vi "Register PVs.vi"(8 "error in (no error)":errorcluster, 10 "Register Info":T1, 11 "CS++PVMonitor in":refnum<class "CS++PVMonitor.lvclass">) -> (0 "error out":errorcluster, 3 "CS++PVMonitor out":refnum<class "CS++PVMonitor.lvclass">)   [LabVIEW 2015, in "CS++PVMonitor.lvlib" / "CS++PVMonitor.lvclass"]
doc: "Register value change monitoring for process variables."
uses:
  CS++PVMonitor.lvclass
  <vilib>/ActorFramework/Message Enqueuer/Message Enqueuer.lvclass
  CS++PVMonitor Messages/CS++PVUpdate Msg/CS++PVUpdate Msg.lvclass
  CS++PVMonitor Messages/CS++PVUpdate Msg/CS++PVUpdate Msg.lvclass/CS++PVUpdate Msg.ctl
  CS++PVMonitor.lvclass/CS++PVMonitor.ctl
  Classes/CS++ProcessVariables/ProcessVariable/PV.lvclass/PV.ctl
  Classes/CS++ProcessVariables/ProcessVariable/PV.lvclass
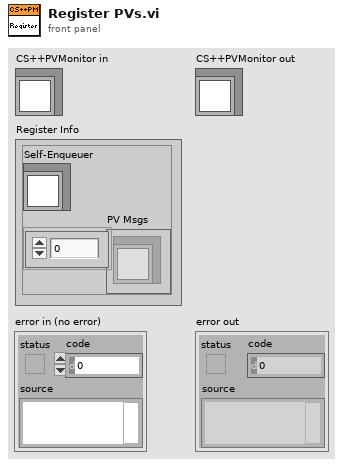
[diagram p1: front panel]
types:
  T1 = cluster{"Self-Enqueuer":refnum<class "Message Enqueuer.lvclass">, "PV Msgs":refnum<class "CS++PVUpdate Msg.lvclass">[]}
  T2 = cluster{"PV URL":string, "Observers":cluster{"Enqueuer":refnum<class "Message Enqueuer.lvclass">, "CS++PVUpdate Msg":refnum<class "CS++PVUpdate Msg.lvclass">}[]}[]
  T3 = cluster{"PV URL":string, "Observers":cluster{"Enqueuer":refnum<class "Message Enqueuer.lvclass">, "CS++PVUpdate Msg":refnum<class "CS++PVUpdate Msg.lvclass">}[]}
  T4 = cluster{"Enqueuer":refnum<class "Message Enqueuer.lvclass">, "CS++PVUpdate Msg":refnum<class "CS++PVUpdate Msg.lvclass">}[]
  T5 = cluster{"Self-Enqueuer":refnum<class "Message Enqueuer.lvclass">, "CS++PVUpdate Msg":refnum<class "CS++PVUpdate Msg.lvclass">}
  T6 = cluster{"Self-Enqueuer":refnum<class "Message Enqueuer.lvclass">, "CS++PVUpdate Msg":refnum<class "CS++PVUpdate Msg.lvclass">}[]
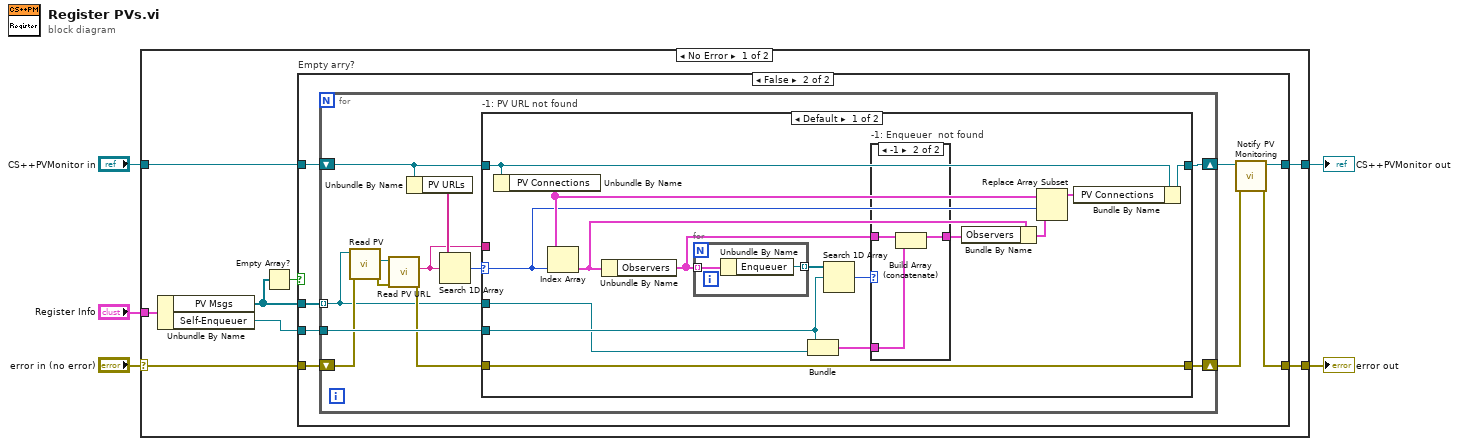
[diagram p0: block diagram]
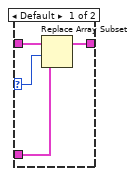
[diagram p3: hidden frame]
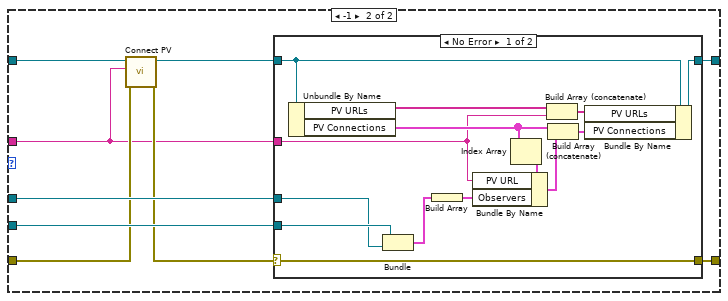
[diagram p4: hidden frame]
diagram:
  n1 = case shown="No Error" "error in (no error)" {
    selector: "error in (no error)" -> [w12 w86]
    tunnel: [w11 w86] -> w4
    tunnel: [w9 w85] -> w2
    tunnel: "CS++PVMonitor in" -> [w10 w85]
    tunnel: "Register Info" -> [w13 _]
    frame No Error {
      n2 = Unbundle By Name(w13) -> ("PV Msgs"=w6:refnum<class "CS++PVUpdate Msg.lvclass">[], "Self-Enqueuer"=w8:refnum<class "Message Enqueuer.lvclass">)
      n3 = Empty Array?(array=w6) -> (empty?=w7:bool)
      n4 = case "Empty arry?" shown="False" w7 {
        tunnel: w6 -> [_ w23]
        tunnel: w12 -> [w14 w22]
        tunnel: [w14 w16] -> w11
        tunnel: w10 -> [w15 w21]
        tunnel: [w15 w18] -> w9
        tunnel: w8 -> [_ w20]
        frame True {
        }
        frame False {
          n5 = for {
            tunnel: w23 -> [w24] mode=indexing
            shift-right: [w30] -> w17
            shift-left: w22 -> [w26]
            shift-right: [w31] -> w19
            shift-left: w21 -> [w33]
            tunnel: w20 -> [w32]
            n6 = call "Read PV.vi"("error in (no error)"=w26, "CS++PVUpdate Msg in"=w24) -> ("error out"=w28:errorcluster, "PV"=w29:refnum<class "PV.lvclass">)  [unwired: 7 in, 1 out]
            n7 = call "Read PV URL.vi"("error in (no error)"=w28, "PV in"=w29) -> ("error out"=w25:errorcluster, "PV URL"=w27:string)  [unwired: 7 in, 1 out]
            n8 = Unbundle By Name(w33) -> ("PV URLs"=w35:string[])
            n9 = Search 1D Array(1D array=w35, element=w27) -> (index of element=w34:i32)  [unwired: 1 in]
            n10 = case "-1: PV URL not found" shown="Default" w34 {
              selector: w34 -> [w45 _]
              tunnel: w33 -> [w49 w64]
              tunnel: w32 -> [w42 w67]
              tunnel: w24 -> [w36 w66]
              tunnel: [w47 w68] -> w31
              tunnel: [w44 w65] -> w30
              tunnel: w25 -> [w44 w62]
              tunnel: w27 -> [_ w60]
              frame Default {
                n11 = Unbundle By Name(w49) -> ("PV Connections"=w46:T2)
                n12 = Index Array(array=w46, index=w45) -> (element=w43:T3)
                n13 = Unbundle By Name(w43) -> ("Observers"=w48:T4)
                n14 = for {
                  tunnel: w48 -> [w59] mode=indexing
                  tunnel: [w58] -> w50 mode=indexing
                  n15 = Unbundle By Name(w59) -> ("Enqueuer"=w58:refnum<class "Message Enqueuer.lvclass">)
                }
                n16 = Bundle("Self-Enqueuer"=w42, "CS++PVUpdate Msg"=w36) -> (w41:T5)  [unwired: 1 in]
                n17 = Search 1D Array(1D array=w50, element=w42) -> (index of element=w37:i32)  [unwired: 1 in]
                n18 = case "-1: Enqueuer  not found" shown="-1" w37 {
                  selector: w37 -> [w51 _]
                  tunnel: w48 -> [w54 w57]
                  tunnel: w41 -> [w53 w55]
                  tunnel: [w52 w56] -> w39
                  frame Default {
                    n19 = Replace Array Subset(array=w54, new element=w53, index=w51) -> (w52:T4)
                  }
                  frame -1 {
                    n20 = Build Array (concatenate)(w57, w55) -> (w56:T6)
                  }
                }
                n21 = Bundle By Name(cluster=w43, "Observers"=w39) -> (w38:T3)
                n22 = Replace Array Subset(array=w46, new element=w38, index=w45) -> (w40:T2)
                n23 = Bundle By Name(cluster=w49, "PV Connections"=w40) -> (w47:refnum<class "CS++PVMonitor.lvclass">)
              }
              frame -1 {
                n24 = call-dynamic "Connect PV.vi"("error in (no error)"=w62, "PV URL"=w60, "CS++PVMonitor in"=w64) -> ("error out"=w61:errorcluster, "CS++PVMonitor out"=w63:refnum<class "CS++PVMonitor.lvclass">)  [unwired: 7 in]
                n25 = case shown="No Error" w61 {
                  selector: w61 -> [w70 w83]
                  tunnel: [w82 w84] -> w68
                  tunnel: w67 -> [w79 _]
                  tunnel: w66 -> [w69 _]
                  tunnel: w63 -> [w74 w84]
                  tunnel: w60 -> [w72 _]
                  tunnel: [w70 w83] -> w65
                  frame No Error {
                    n26 = Unbundle By Name(w74) -> ("PV URLs"=w71:string[], "PV Connections"=w81:T2)
                    n27 = Bundle("Self-Enqueuer"=w79, "CS++PVUpdate Msg"=w69) -> (w78:T5)  [unwired: 1 in]
                    n28 = Build Array(w78) -> (w76:T6)
                    n29 = Index Array(array=w81) -> (element=w80:T3)  [unwired: 1 in]
                    n30 = Bundle By Name(cluster=w80, "PV URL"=w72, "Observers"=w76) -> (w75:T3)
                    n31 = Build Array (concatenate)(w71, w72) -> (w73:string[])
                    n32 = Build Array (concatenate)(w81, w75) -> (w77:T2)
                    n33 = Bundle By Name(cluster=w74, "PV URLs"=w73, "PV Connections"=w77) -> (w82:refnum<class "CS++PVMonitor.lvclass">)
                  }
                  frame Error {
                  }
                }
              }
            }
          }
          n34 = call-dynamic "Notify PV Monitoring.vi"("error in (no error)"=w17, "CS++PVMonitor in"=w19) -> ("error out"=w16:errorcluster, "CS++PVMonitor out"=w18:refnum<class "CS++PVMonitor.lvclass">)  [unwired: 8 in]
        }
      }
    }
    frame Error {
    }
  }
  "error out" <- w4
  "CS++PVMonitor out" <- w2
